vi "Sea-Level SWI Install.vi"() -> ()   [LabVIEW 2011]
panel:
  out "error out":errorcluster
  in  "error in (no error)":errorcluster
  in  "FILE":string
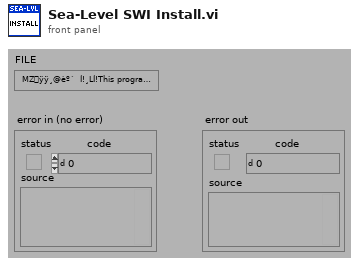
[diagram p1: front panel]
types:
  T1 = enum16{"open", "replace", "create", "open or create", "replace or create", "replace or create with confirmation"}
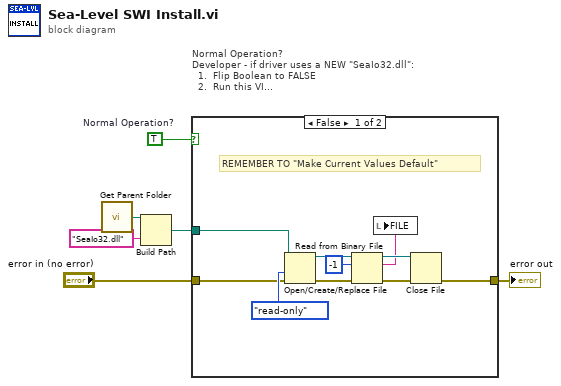
[diagram p0: block diagram]
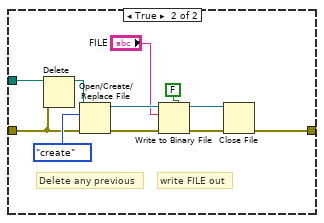
[diagram p2: hidden frame]
diagram:
  w2 = TRUE  # Normal Operation?
  n1 = call "Get Parent Folder.vi"() -> ("path"=w6:path)  [unwired: 5 out]
  n2 = Build Path(base path=w6, name or relative path="SeaIo32.dll") -> (appended path=w4:path)
  n3 = case "Normal Operation?\nDeveloper - if driver uses a NEW \"SeaIo32.dll\":\n  1.  Flip Boolean to FALSE\n  2.  Run this VI\n  3.  Flip Boolean back to TRUE\n  4.  Edit >> \"Make Current Values Default\" and Save the VI" shown="False" w2 {
    tunnel: w4 -> [w9 w19]
    tunnel: [w7 w18] -> w3
    tunnel: "error in (no error)" -> [w10 w17]
    frame False {
      # "REMEMBER TO \"Make Current Values Default\""
      n4 = Open/Create/Replace File(file path (use dialog)=w9, error in=w10, access (0:read/write)=enum16{"read/write", "read-only", "write-only"}."read-only") -> (refnum out=w12:refnum<file>, error out=w11:errorcluster)  [unwired: 4 out]
      n5 = Read from Binary File(8:w11, 10:-1 ("count (1)"), 11:w12) -> (0:w14:errorcluster, 2:w8:string, 3:w15:refnum<file>)  [unwired: 4 out]
      n6 = local write "FILE"(w8) -> ()
      n7 = Close File(refnum=w15, error in=w14) -> (error out=w7:errorcluster)  [unwired: 1 out]
    }
    frame True {
      # "write FILE out"
      # "Delete any previous"
      n8 = Delete(path (use dialog)=w19, error in=w17) -> (deleted path=w20:path)  [unwired: 5 out]
      n9 = Open/Create/Replace File(file path (use dialog)=w20, error in=w17, operation (0:open)=T1."create") -> (refnum out=w24:refnum<file>, error out=w23:errorcluster)  [unwired: 4 out]
      n10 = Write to Binary File(file (use dialog)=w24, data="FILE", error in=w23, 5:FALSE ("prepend array or string size? (T)")) -> (refnum out=w26:refnum<file>, error out=w27:errorcluster)  [unwired: 3 out]
      n11 = Close File(refnum=w26, error in=w27) -> (error out=w18:errorcluster)  [unwired: 1 out]
    }
  }
  "error out" <- w3
